vi "Select spot to transform.vi"(0 "TopLevelDataFilePath":path=path "/INL Macintosh/Users/timothymcjunkin/Documents/First_round_samples_FY2011_Test/Sample_9 Karens Granite/Karens granite session 4 session5 session6/Karens granite session4 session5 comparison.xml", 1 "Sample Information":T4={"Sample Name/ID"="Diffusion_sample", "Notes on Sample"="", "Session_list"=[{"Instrument"=2, "Session_data_base"=path "/INL Macintosh/Users/timothymcjunkin/Desktop/Diffusion couple/JEOL 7000F SEM 9-3-10/Jeol_9-3-10.xml", "Session Name/ID"="Initial Joel location"}, {"Instrument"=3, "Session_data_base"=path "/INL Macintosh/Users/timothymcjunkin/Desktop/Diffusion couple/MXRD 9-13-10/xrd_session.xlm", "Session Name/ID"="xrd_test"}, {"Instrument"=2, "Session_data_base"=path "/INL Macintosh/Users/timothymcjunkin/Desktop/Diffusion couple/JEOL 7000F SEM 9-3-10/Corrected_9-3-10.xlm", "Session Name/ID"="Correct_Abs_position"}]} {"Session_list"."Instrument" items=["Unknown", "Phillips SEM IRC", "JEOL 7000F EML_MFC", "MXRD MFC", "JEOL_EPMA"]}, 2 "Current Session Information":T1, 3 "PositionFromPreviousSession":u16(ring) items=["Fid3", "POI2", "Fiducial5", "POI1", "POI1-alt"], 4 "RefernceSessionInput":i32) -> (5 "SelectedSpotInfo":T2, 6 "Cancel out":bool)   [LabVIEW 2011]
doc: "This dialog box is displayed when the user selects \"Find A Point from a Previous Session\" button on the main user interface. This dialog box gives the user the ability to choose from a list of points that can be transformed from a selected previous session. The list will contain the points that may be transformed from the selected session. The user may change the selected session from which to transform. All prior sessions are displayed even though the are not guaranteed to have enough matching fiducials to produce a transformation. [A future revision of the software may check for this and limit the list of sessions to those that are viable] When a session and/or point is chosen the form will display the information for the point to be transformed. The user may at anytime press cancel to exit without adding a transformed point or hit OK to continue to the next step in adding the point to the database. This dialog box does not have the capability to edit notes or coordinates. The next dialog box in the process of adding a point will have that capability."
uses:
  cm2nm_sample_set.ctl
  cm2nm_coordinate_information_v2.ctl
  Instrument_type_enum_v2.ctl
panel:
  out "FidcucialMetrics":cluster{"M1":dbl, "M2":dbl, "S1":dbl, "S2":dbl}
  out "Current Session Information_inloop":T1 caption="Current Session Information"
  out "Collection without calculated points.":T2[](array[typedef])
  out "Indices of calculated positions":i32[](array[numeric])
  in  "Reference Session":u16(ring) items=["Session_1_JEOL_7000", "Session_2_MXRD", "Session_3_EML_FIB"]
  in  "Cancel":bool
  in  "OK":bool
  # "Select a different\nReference Session"
  # "Select a spot\nthat you would\nlike to find\nin the current\nsession.\n\nThen Press\nOK."
  # "This form\ndisplay the\ninformation\nabout the\nchosen\nposition"
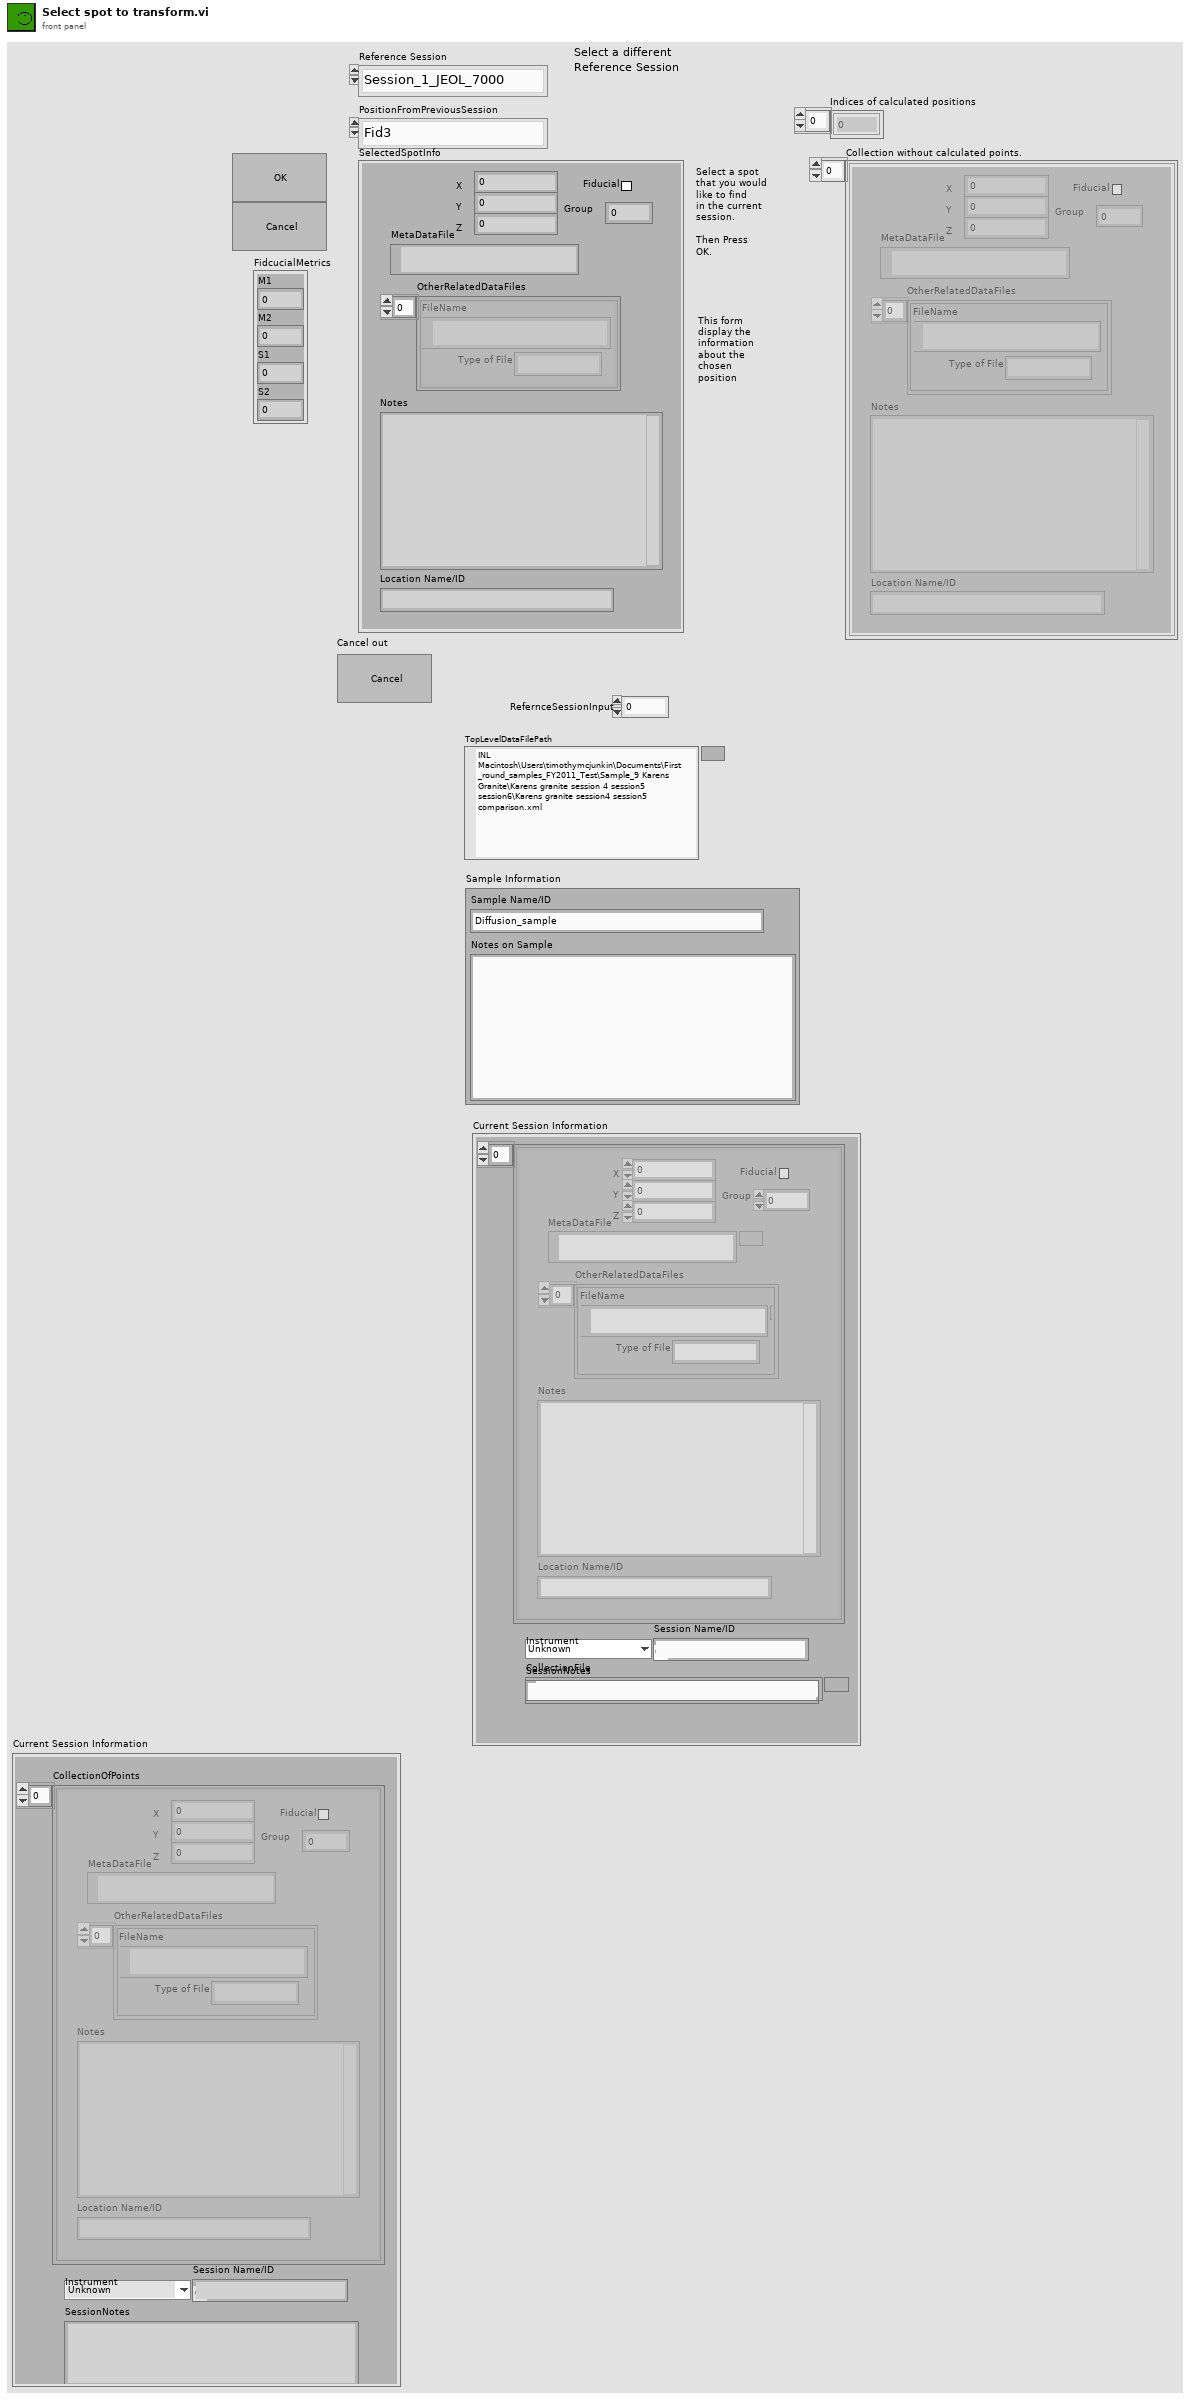
[diagram p1: front panel]
types:
  T1 = typedef "cm2nm_sample_set.ctl" = cluster{"CollectionOfPoints":T2[], "Instrument":T3, "CollectionFile":path, "Session Name/ID":string, "SessionNotes":string}
  T2 = typedef "cm2nm_coordinate_information_v2.ctl" = cluster{"MetaDataFile":path, "X":dbl, "Y":dbl, "Z":dbl, "Group":i32, "Rotation":dbl[unit], "Fiducial":bool, "Magnification":dbl, "Working_Distance":dbl, "Notes":string, "Location Name/ID":string, "OtherRelatedDataFiles":cluster{"Type of File":string, "FileName":path}[], "Available":bool}
  T3 = typedef "Instrument_type_enum_v2.ctl" = enum16{"Unknown", "Philips FEI SEM IRC", "JEOL 7000F EML_MFC", "MXRD MFC", "JEOL_EPMA"}
  T4 = cluster{"Sample Name/ID":string, "Notes on Sample":string, "Session_list":cluster{"Instrument":u16, "Session_data_base":path, "Session Name/ID":string}[]}
  T5 = enum8{"Enabled", "Disabled", "Disabled and Grayed Out"}
  T6 = cluster{"Instrument":u16, "Session_data_base":path, "Session Name/ID":string}[]
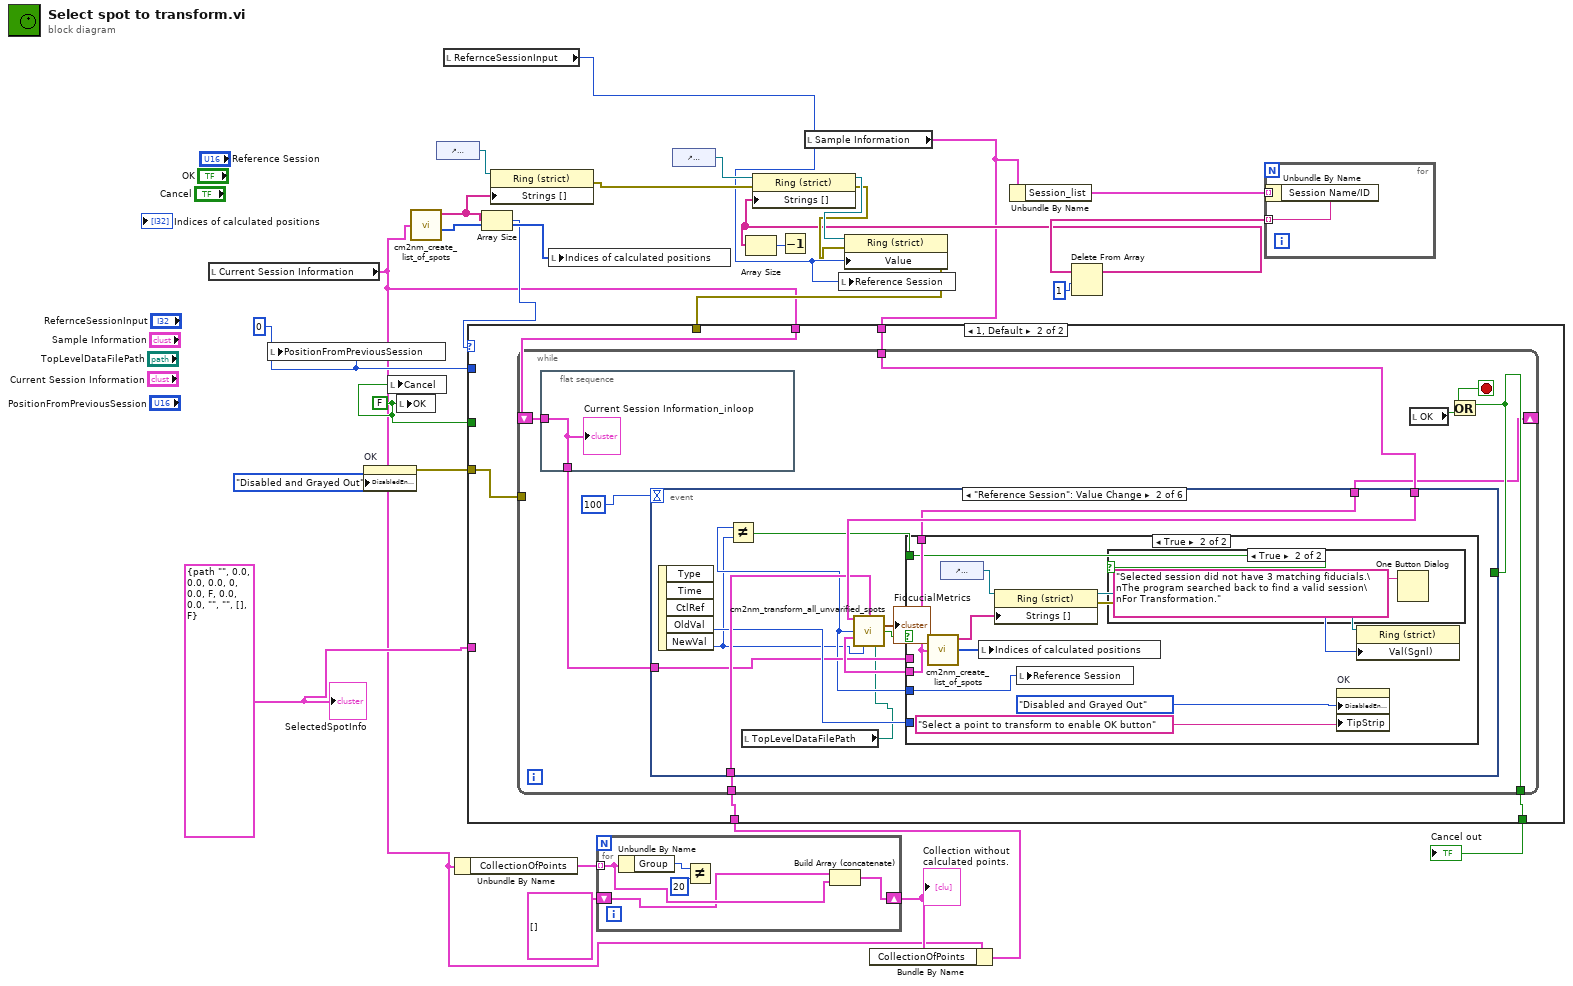
[diagram p0: block diagram]
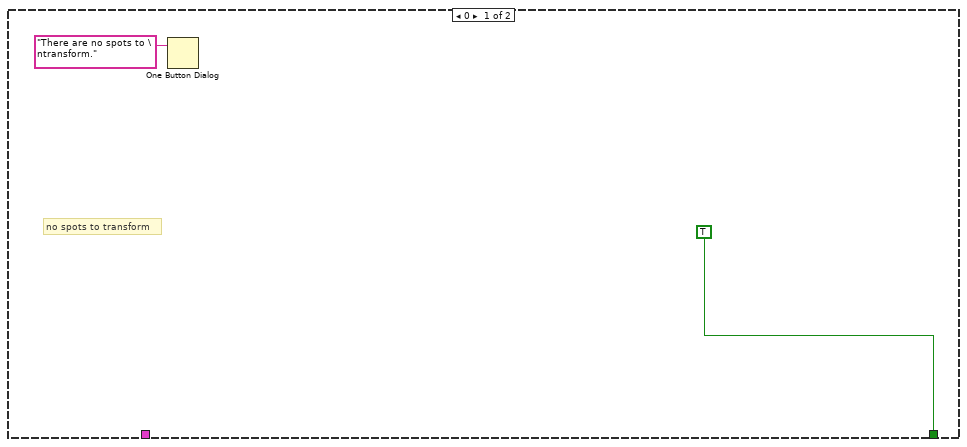
[diagram p2: hidden frame]
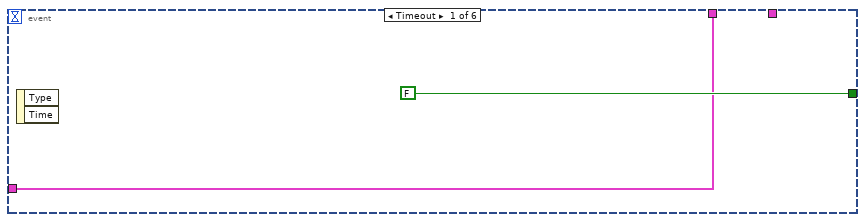
[diagram p3: hidden frame]
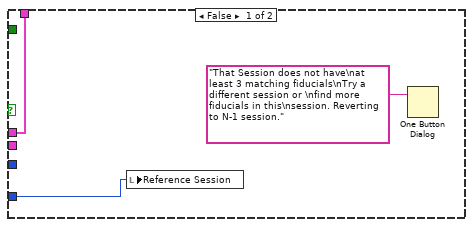
[diagram p4: hidden frame]
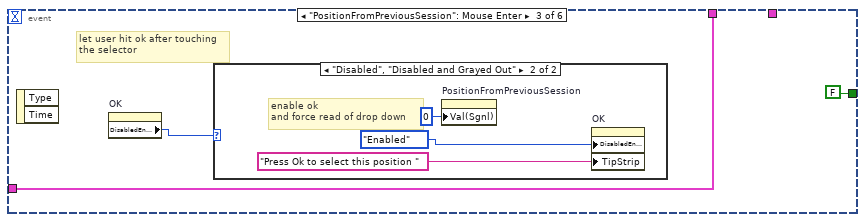
[diagram p6: hidden frame]
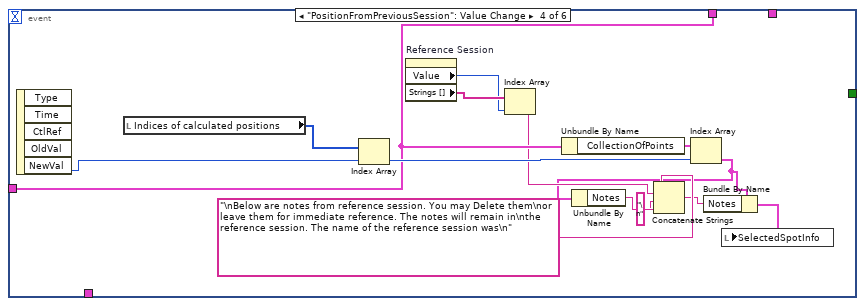
[diagram p8: hidden frame]
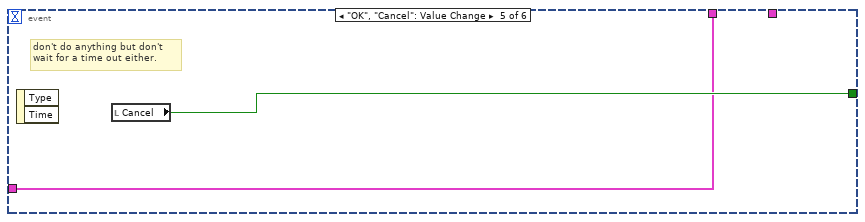
[diagram p9: hidden frame]
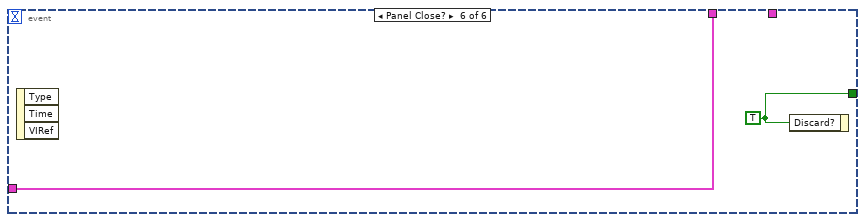
[diagram p10: hidden frame]
diagram:
  w4 = T2 {"MetaDataFile"=path "", "X"=0.0, "Y"=0.0, "Z"=0.0, "Group"=0, "Rotation"=0.0, "Fiducial"=FALSE, "Magnification"=0.0, "Working_Distance"=0.0, "Notes"="", "Location Name/ID"="", "OtherRelatedDataFiles"=[], "Available"=FALSE} ("SelectedSpotInfo")
  w23 = 0
  w24 = FALSE ("OK")
  n1 = local read "Current Session Information"() -> (w1:T1)
  n2 = local write "PositionFromPreviousSession"(w23) -> ()
  n3 = property on="OK" class="Bool (strict)"("DisabledEnum"=T5."Disabled and Grayed Out" ("Disabled")) -> (error out=w26:errorcluster)  [unwired: 2 in, 1 out]
  n4 = local write "Cancel"(w24) -> ()
  n5 = local write "OK"(w24) -> ()
  n6 = call "cm2nm_create_list_of_spots.vi"("Current Session"=w1) -> ("Indices of calculated positions"=w7:i32[], "Name of calculated positions"=w8:string[])  [unwired: 2 out]
  n7 = control-ref of="PositionFromPreviousSession"() -> (w9:refnum<vi>)
  n8 = local read "RefernceSessionInput"() -> (w3:i32)
  n9 = Unbundle By Name(w1) -> ("CollectionOfPoints"=w13:T2[])
  n10 = Array Size(array=w8) -> (size(s)=w6:i32)
  n11 = property on="Property Node" class="Ring (strict)"(reference=w9, "Strings []"=w8) -> (error out=w5:errorcluster)  [unwired: 1 in, 1 out]
  n12 = local write "Indices of calculated positions"(w7) -> ()
  n13 = for {
    tunnel: w13 -> [w30] mode=indexing
    shift-right: [w29] -> w11
    shift-left: T2[] [] -> [w28]
    n14 = Unbundle By Name(w30) -> ("Group"=w32:i32)
    n15 = Not Equal?(x=w32, y=20) -> ()  [unwired: 1 out]
    n16 = Build Array (concatenate)(w28, w30) -> (w29:T2[])
  }
  "Collection without calculated points." <- w11
  n17 = control-ref of="Reference Session"() -> (w22:refnum<vi>)
  n18 = local read "Sample Information"() -> (w2:T4)
  n19 = local write "Reference Session"(w3) -> ()
  n20 = Bundle By Name(cluster=w1, "CollectionOfPoints"=w11) -> (w10:T1)
  n21 = Unbundle By Name(w2) -> ("Session_list"=w14:T6)
  n22 = for {
    tunnel: w14 -> [w34] mode=indexing
    tunnel: [w33] -> w21 mode=indexing
    n23 = Unbundle By Name(w34) -> ("Session Name/ID"=w33:string)
  }
  n24 = Delete From Array(array=w21, length=1) -> (array with subset deleted=w16:string[])  [unwired: 1 in, 1 out]
  n25 = Array Size(array=w16) -> (size(s)=w15:i32)
  n26 = property on="Property Node" class="Ring (strict)"(reference=w22, error in=w5, "Strings []"=w16) -> (reference out=w19:refnum<vi>, error out=w18:errorcluster)
  n27 = Decrement(x=w15) -> ()  [unwired: 1 out]
  n28 = property on="Property Node" class="Ring (strict)"(reference=w19, error in=w18, "Value"=w3) -> (error out=w17:errorcluster)  [unwired: 1 out]
  n29 = case shown="1, Default" w6 {
    tunnel: w1 -> [_ w37]
    tunnel: w26 -> [_ w41]
    tunnel: [TRUE ("Cancel") w40] -> w25
    tunnel: w24 -> [_ _]
    tunnel: w23 -> [_ _]
    tunnel: w17 -> [_ _]
    tunnel: w2 -> [_ w39]
    tunnel: w10 -> [_ w38]
    tunnel: w4 -> [_ _]
    frame 0 {
      # "no spots to transform"
      n30 = One Button Dialog(message="There are no spots to \ntransform.") -> ()  [unwired: 1 in, 1 out]
    }
    frame 1, Default {
      n31 = while {
        tunnel: w41 -> [_]
        tunnel: [w47] -> w40
        tunnel: w39 -> [w46]
        tunnel: w38 -> [w45]
        shift-right: [w43] -> _
        shift-left: w37 -> [w44]
        stop <- w49 stop-if-true
        n32 = flat-sequence {
          tunnel: w44 -> [w51]
          tunnel: [w51] -> w42
          frame #0 {
            "Current Session Information_inloop" <- w51
          }
        }
        n33 = event shown="[1] \"Reference Session\": Value Change" {
          selector: _ -> [_ _ _ _ _ _]
          dyn-events: _ -> [_ _ _ _ _ _]
          timeout: u32 100 ("millisecond multiple") -> [_ _ _ _ _ _]
          tunnel: [FALSE _ FALSE _ w103 w105] -> w47
          tunnel: w46 -> [_ w65 _ _ _ _]
          tunnel: w45 -> [_ w64 _ _ _ _]
          tunnel: w42 -> [w52 w59 w83 w97 w102 w104]
          tunnel: [w52 w61 w83 w97 w102 w104] -> w43
          event Timeout {
            n34 = event-data() -> ()  [unwired: 1 in, 2 out]
          }
          event "Reference Session": Value Change {
            n35 = event-data() -> ("OldVal"=w60:u16, "NewVal"=w57:u16)  [unwired: 1 in, 3 out]
            n36 = local read "TopLevelDataFilePath"() -> (w55:path)
            n37 = call "cm2nm_transform_all_unvarified_spots.vi"("Sample_Information"=w65, "Current Session Information IN"=w64, "ReferenceSessionIndex"=w57, "TopLevelDataFilePath"=w55) -> ("FidcucialMetrics"=→"FidcucialMetrics":cluster{"M1":dbl, "M2":dbl, "S1":dbl, "S2":dbl}, "CurrentRefSessionIdx"=w58:i32, "OK_num_fids?"=w63:bool, "Current Session InformationOUT"=w62:T1)  [unwired: 1 in, 7 out]
            n38 = Not Equal?(x=w58, y=w57) -> (x != y?=w56:bool)
            n39 = case shown="True" w63 {
              tunnel: w62 -> [_ w77]
              tunnel: [w67 w77] -> w61
              tunnel: w60 -> [w68 _]
              tunnel: w59 -> [w67 _]
              tunnel: w58 -> [_ w71]
              tunnel: w56 -> [_ w69]
              frame False {
                n40 = local write "Reference Session"(w68) -> ()
                n41 = One Button Dialog(message="That Session does not have\nat least 3 matching fiducials\nTry a different session or \nfind more fiducials in this\nsession. Reverting to N-1 session.") -> ()  [unwired: 1 in, 1 out]
              }
              frame True {
                n42 = call "cm2nm_create_list_of_spots.vi"("Current Session"=w77) -> ("Indices of calculated positions"=w80:i32[], "Name of calculated positions"=w79:string[])  [unwired: 2 out]
                n43 = control-ref of="PositionFromPreviousSession"() -> (w78:refnum<vi>)
                n44 = local write "Indices of calculated positions"(w80) -> ()
                n45 = property on="Property Node" class="Ring (strict)"(reference=w78, "Strings []"=w79) -> (reference out=w75:refnum<vi>, error out=w74:errorcluster)  [unwired: 1 in]
                n46 = local write "Reference Session"(w71) -> ()
                n47 = case shown="True" w69 {
                  frame False {
                  }
                  frame True {
                    n48 = One Button Dialog(message="Selected session did not have 3 matching fiducials.\nThe program searched back to find a valid session\nFor Transformation.") -> ()  [unwired: 1 in, 1 out]
                  }
                }
                n49 = property class="Ring (strict)"(reference=w75, error in=w74) -> (reference out=w73:refnum<vi>, "Value"=w72:u16)  [unwired: 1 out]
                n50 = property on="OK" class="Bool (strict)"("DisabledEnum"=T5."Disabled and Grayed Out" ("Disabled"), "TipStrip"="Select a point to transform to enable OK button" ("Tip Strip")) -> ()  [unwired: 2 in, 2 out]
                n51 = property class="Ring (strict)"(reference=w73, "Val(Sgnl)"=w72) -> ()  [unwired: 1 in, 2 out]
              }
            }
          }
          event "PositionFromPreviousSession": Mouse Enter {
            # "let user hit ok after touching\nthe selector"
            n52 = event-data() -> ()  [unwired: 1 in, 2 out]
            n53 = property on="OK" class="Bool (strict)"() -> ("DisabledEnum"=w82:T5)  [unwired: 2 in, 2 out]
            n54 = case shown="\"Disabled\", \"Disabled and Grayed Out\"" w82 {
              frame "Enabled", Default {
              }
              frame "Disabled", "Disabled and Grayed Out" {
                # "enable ok\nand force read of drop down"
                n55 = property on="PositionFromPreviousSession" class="Ring (strict)"("Val(Sgnl)"=u16 0 ("Value (Signaling)")) -> ()  [unwired: 2 in, 2 out]
                n56 = property on="OK" class="Bool (strict)"("DisabledEnum"=T5."Enabled" ("Disabled"), "TipStrip"="Press Ok to select this position " ("Tip Strip")) -> ()  [unwired: 2 in, 2 out]
              }
            }
          }
          event "PositionFromPreviousSession": Value Change {
            n57 = event-data() -> ("NewVal"=w98:u16)  [unwired: 1 in, 4 out]
            n58 = local read "Indices of calculated positions"() -> (w101:i32[])
            n59 = Index Array(array=w101, index=w98) -> (element=w99:i32)
            n60 = property on="Reference Session" class="Ring (strict)"() -> ("Value"=w94:u16, "Strings []"=w95:string[])  [unwired: 2 in, 2 out]
            n61 = Index Array(array=w95, index=w94) -> (element=w92:string)
            n62 = Unbundle By Name(w97) -> ("CollectionOfPoints"=w100:T2[])
            n63 = Index Array(array=w100, index=w99) -> (element=w91:T2)
            n64 = Unbundle By Name(w91) -> ("Notes"=w96:string)
            n65 = Concatenate Strings("\nBelow are notes from reference session. You may Delete them\nor leave them for immediate reference. The notes will remain in\nthe reference session. The name of the reference session was\n", w92, "\n" ("string"), w96) -> (w90:string)
            n66 = Bundle By Name(cluster=w91, "Notes"=w90) -> (w88:T2)
            n67 = local write "SelectedSpotInfo"(w88) -> ()
          }
          event "OK", "Cancel": Value Change {
            # "don't do anything but don't\nwait for a time out either."
            n68 = event-data() -> ()  [unwired: 1 in, 2 out]
            n69 = local read "Cancel"() -> (w103:bool)
          }
          event Panel Close? {
            w105 = TRUE ("Discard?")
            n70 = event-data() -> ()  [unwired: 1 in, 3 out]
            n71 = event-data("Discard?"=w105) -> ()  [unwired: 1 in, 1 out]
          }
        }
        n72 = local read "OK"() -> (w48:bool)
        n73 = Or(x=w47, y=w48) -> (x .or. y?=w49:bool)
      }
    }
  }
  "Cancel out" <- w25
  "SelectedSpotInfo" <- w4
